vi "图片编辑.vi"() -> ()   [LabVIEW 2018]
panel:
  in  "字符串 5":string
  in  "字符串 4":string
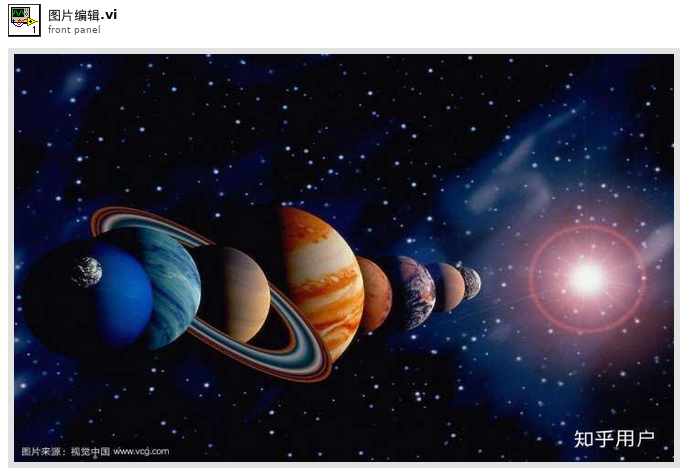
[diagram p1: front panel]
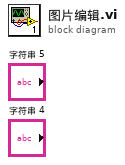
[diagram p0: block diagram]
diagram:
